vi "rd_data (Array of DBL).vi"(4 "record index":u32, 6 "record info":T3, 7 "recordLenFromStart":u64, 8 "error in (no error)":errorcluster, 9 "length":u64, 10 "record start":u64, 11 "ExcelRefnum":T4) -> (0 "error out":errorcluster, 2 "data_AllTypeData":T1, 3 "real length":u64)   [LabVIEW 2020, in "NI_ExcelFile.lvlib"]
uses:
  <vilib>/express/express shared/NI_ExcelFile/NI_ExcelFile.lvlib
  <vilib>/express/express shared/NI_ExcelFile/Ctrls/ExcelRefnum.ctl
  <vilib>/express/express shared/NI_ExcelFile/Ctrls/MainData.ctl
  <vilib>/express/express shared/NI_ExcelFile/Ctrls/StreamMode.ctl
  <vilib>/express/express shared/NI_ExcelFile/Ctrls/TimeColumnMode.ctl
  <vilib>/express/express shared/NI_ExcelFile/Ctrls/FileAttribute.ctl
  <vilib>/express/express shared/NI_ExcelFile/Ctrls/Columns.ctl
  <vilib>/express/express shared/NI_ExcelFile/Ctrls/ColumnInfo.ctl
  <vilib>/express/express shared/NI_ExcelFile/Ctrls/DataType.ctl
  <vilib>/express/express shared/NI_ExcelFile/Ctrls/wd_recordInfo.ctl
  <vilib>/express/express shared/NI_ExcelFile/Ctrls/disk_TemplateFile.ctl
  <vilib>/express/express shared/NI_ExcelFile/Ctrls/meta_file.ctl
  <vilib>/express/express shared/NI_ExcelFile/Ctrls/meta_Block.ctl
  <vilib>/express/express shared/NI_ExcelFile/Ctrls/meta_BlockType.ctl
  <vilib>/express/express shared/NI_ExcelFile/Ctrls/data_AllTypeData.ctl
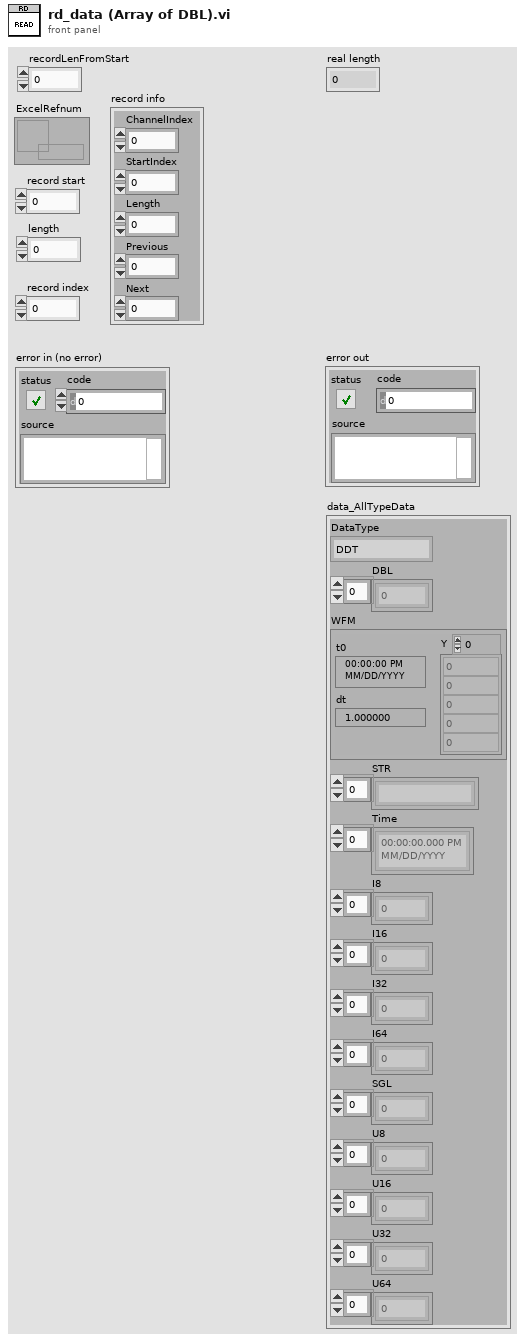
[diagram p1: front panel]
types:
  T1 = typedef "NI_ExcelFile.lvlib/data_AllTypeData.ctl" = cluster{"DataType":T2, "DBL":dbl[], "WFM":waveform(dbl), "STR":string[], "Time":timestamp[], "I8":i8[], "I16":i16[], "I32":i32[], "I64":i64[], "SGL":sgl[], "U8":u8[], "U16":u16[], "U32":u32[], "U64":u64[]}
  T2 = typedef "NI_ExcelFile.lvlib/DataType.ctl" = enum16{"DDT", "WFM", "Array of STR", "Array of DBL", "Array of I8", "Array of I16", "Array of I32", "Array of I64", "Array of SGL", "Array of U8", "Array of U16", "Array of U32", "Array of U64", "Array of Time"}
  T3 = typedef "NI_ExcelFile.lvlib/wd_recordInfo.ctl" = cluster{"ChannelIndex":u32, "StartIndex":u64, "Length":u64, "Previous":i32, "Next":i32}
  T4 = typedef "NI_ExcelFile.lvlib/ExcelRefnum.ctl" = refnum<data-value>
  T5 = typedef "NI_ExcelFile.lvlib/MainData.ctl" = cluster{"TargetFile":path, "StreamMode":T6, "Append?":bool, "ChunkSize":u64, "TimeColumnMode":T7, "TimestampFormat":string, "AbsoluteTime?":bool, "FileAttribute ":T8, "Column":T9, "FileRef":refnum<k1>, "MemoryRef":refnum<data-value>[], "RecordInfo":T3[], " ChannelPreviousInfo":u32[], "ChannelFirstRecord":u32[], "PredefinedFormattedValueLength":i64, "DiskTemplate":T11}
  T6 = typedef "NI_ExcelFile.lvlib/StreamMode.ctl" = enum16{"File", "Memory"}
  T7 = typedef "NI_ExcelFile.lvlib/TimeColumnMode.ctl" = enum16{"Empty", "OnePerCh", "One"}
  T8 = typedef "NI_ExcelFile.lvlib/FileAttribute.ctl" = cluster{"Creator":string, "Title":string, "SheetName":string}
  T9 = typedef "NI_ExcelFile.lvlib/Columns.ctl" = T10[]
  T10 = typedef "NI_ExcelFile.lvlib/ColumnInfo.ctl" = cluster{"Header":string, "Format":string, "DataType":T2, "Length":u64}
  T11 = typedef "NI_ExcelFile.lvlib/disk_TemplateFile.ctl" = cluster{"XMLRef":refnum<file>[], "ZipPath":path, "MetaFile":T12, "TempFolder":path}
  T12 = typedef "NI_ExcelFile.lvlib/meta_file.ctl" = cluster{"Ref":refnum<file>, "NextRow":i32, "NextPosition":i64, "Block":T13[]}
  T13 = typedef "NI_ExcelFile.lvlib/meta_Block.ctl" = cluster{"Version":u16, "Type":T14, "Length":i32, "Data":string}
  T14 = typedef "NI_ExcelFile.lvlib/meta_BlockType.ctl" = enum16{"NITag", "File", "Column"}
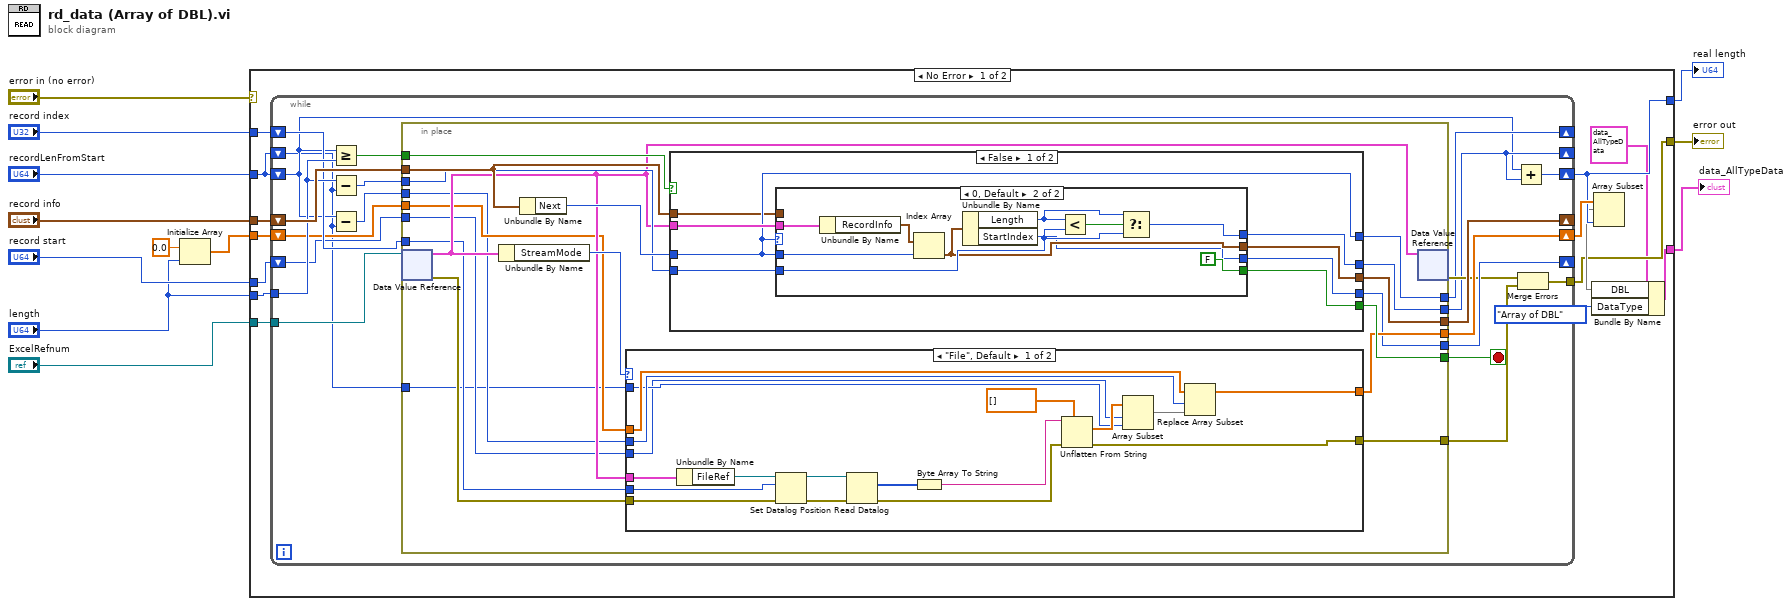
[diagram p0: block diagram]
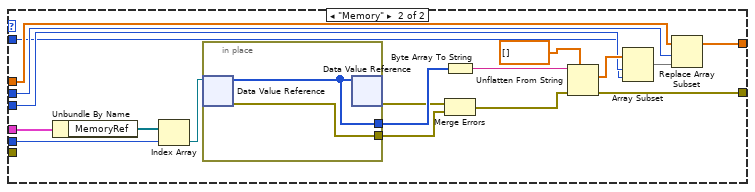
[diagram p2: hidden frame]
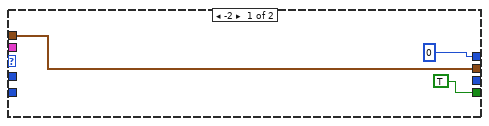
[diagram p3: hidden frame]
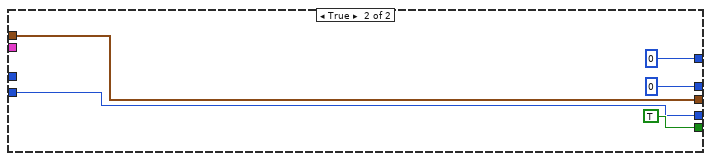
[diagram p4: hidden frame]
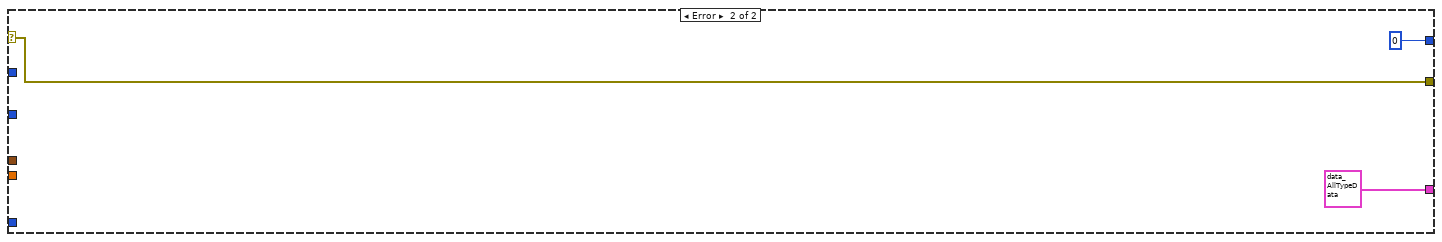
[diagram p5: hidden frame]
diagram:
  n1 = Initialize Array(0.0 ("element"), "length") -> (w3:dbl[])
  n2 = case shown="No Error" "error in (no error)" {
    selector: "error in (no error)" -> [_ w133]
    tunnel: w3 -> [w20 _]
    tunnel: [w15 w133] -> w12
    tunnel: "record start" -> [w26 _]
    tunnel: "record index" -> [w22 _]
    tunnel: "ExcelRefnum" -> [w25 _]
    tunnel: "recordLenFromStart" -> [w21 _]
    tunnel: "length" -> [w24 _]
    tunnel: "record info" -> [w23 _]
    tunnel: [w18 u64 0 ("recordLenFromStart")] -> w6
    tunnel: [w14 T1 {"DataType"=enum."DDT", "DBL"=[], "WFM"={"t0"=timestamp(0 s since 1904-01-01), "dt"=1.0, "Y"=[]}, "STR"=[], "Time"=[], "I8"=[], "I16"=[], "I32"=[], "I64"=[], "SGL"=[], "U8"=[], "U16"=[], "U32"=[], "U64"=[]} ("fmt_AllTypeData")] -> w1
    frame No Error {
      n3 = while {
        shift-right: [w30] -> _
        shift-left: w21 -> [w28]
        tunnel: w24 -> [w44]
        shift-right: [w45] -> _
        shift-left: w23 -> [w46]
        tunnel: w25 -> [w47]
        shift-right: [w42] -> w18
        shift-left: w21 -> [w29]
        shift-right: [w36] -> w19
        shift-left: w20 -> [w37]
        shift-right: [w31] -> _
        shift-left: w22 -> [w40]
        shift-right: [w35] -> _
        shift-left: w26 -> [w39]
        tunnel: [w32] -> w15
        stop <- w38 stop-if-true
        n4 = Greater Or Equal?(x=w29, y=w44) -> (x >= y?=w41:bool)
        n5 = Subtract(x=w44, y=w28) -> (x-y=w43:u64)
        n6 = Subtract(x=w29, y=w28) -> (x-y=w27:u64)
        n7 = in-place {
          in-place-border: w46 -> [w65]
          in-place-border: w28 -> [w48]
          in-place-border: [w63] -> w45
          in-place-border: w43 -> [w62]
          in-place-border: [w61] -> w30
          in-place-border: w41 -> [w60]
          in-place-border: w40 -> [w57]
          in-place-border: w39 -> [w56]
          in-place-border: [w55] -> w31
          in-place-border: [w54] -> w38
          in-place-border: w37 -> [w53]
          in-place-border: [w52] -> w36
          in-place-border: [w51] -> w35
          in-place-border: [w50] -> w33
          in-place-border: w27 -> [w49]
          n8 = in-place-dvr #1(w47) -> (w58:T5, w66:errorcluster)
          n9 = Unbundle By Name(w58) -> ("StreamMode"=w59:T6)
          n10 = Unbundle By Name(w65) -> ("Next"=w64:i32)
          n11 = case shown="\"File\", Default" w59 {
            tunnel: w57 -> [w81 w95]
            tunnel: w66 -> [w80 _]
            tunnel: w56 -> [w67 w92]
            tunnel: w58 -> [w83 w102]
            tunnel: w53 -> [w76 w100]
            tunnel: [w75 w99] -> w52
            tunnel: [w71 w90] -> w50
            tunnel: w49 -> [w69 w86]
            tunnel: w48 -> [w68 w85]
            frame "File", Default {
              n12 = Unbundle By Name(w83) -> ("FileRef"=w82:refnum<k1>)
              n13 = Set Datalog Position(4:w80, 6:w81, 7:w82) -> (0:w79:errorcluster, 3:w84:refnum<k1>)  [unwired: 1 in]
              n14 = Read Datalog(4:w79, 7:w84) -> (0:w72:errorcluster, 2:w78:u8[])  [unwired: 1 in, 1 out]
              n15 = Byte Array To String(unsigned byte array=w78) -> (string=w77:string)
              n16 = Unflatten From String(type=dbl[] [] ("Initial data"), binary string=w77, error in (no error)=w72) -> (value=w73:dbl[], error out=w71:errorcluster)  [unwired: 2 in, 1 out]
              n17 = Array Subset(array=w73, index=w67, length=w68) -> (w70:dbl[])
              n18 = Replace Array Subset(array=w76, new element=w70, index=w69) -> (w75:dbl[])
            }
            frame "Memory" {
              n19 = Unbundle By Name(w102) -> ("MemoryRef"=w96:refnum<data-value>[])
              n20 = Index Array(array=w96, index=w95) -> (element=w94:refnum<data-value>)
              n21 = in-place {
                in-place-border: [w104] -> w93
                in-place-border: [w103] -> w88
                n22 = in-place-dvr #2(w94) -> (w104:u8[], w103:errorcluster)
                n23 = in-place-dvr #2(w104) -> (w91:errorcluster)  [unwired: 1 out]
              }
              n24 = Byte Array To String(unsigned byte array=w93) -> (string=w101:string)
              n25 = Merge Errors(w91, w88) -> (w89:errorcluster)
              n26 = Unflatten From String(type=dbl[] [] ("Initial data"), binary string=w101, error in (no error)=w89) -> (value=w97:dbl[], error out=w90:errorcluster)  [unwired: 2 in, 1 out]
              n27 = Array Subset(array=w97, index=w92, length=w85) -> (w87:dbl[])
              n28 = Replace Array Subset(array=w100, new element=w87, index=w86) -> (w99:dbl[])
            }
          }
          n29 = case shown="False" w60 {
            tunnel: w65 -> [w107 w127]
            tunnel: w64 -> [w108 _]
            tunnel: [w109 w127] -> w63
            tunnel: w62 -> [w110 w126]
            tunnel: [w112 u64 0 ("Length")] -> w61
            tunnel: w58 -> [w111 _]
            tunnel: [w108 u32 0 ("next")] -> w55
            tunnel: [w106 TRUE] -> w54
            tunnel: [w105 w126] -> w51
            frame False {
              n30 = case shown="0, Default" w108 {
                tunnel: [u64 0 ("Length") w123] -> w112
                tunnel: w111 -> [_ w122]
                tunnel: w108 -> [_ w121]
                tunnel: w110 -> [_ w120]
                tunnel: [w115 w119] -> w109
                tunnel: w107 -> [w115 _]
                tunnel: [TRUE FALSE] -> w106
                tunnel: [_ w117] -> w105
                frame -2 {
                }
                frame 0, Default {
                  n31 = Unbundle By Name(w122) -> ("RecordInfo"=w125:T3[])
                  n32 = Index Array(array=w125, index=w121) -> (element=w119:T3)
                  n33 = Unbundle By Name(w119) -> ("Length"=w116:u64, "StartIndex"=w117:u64)
                  n34 = Less?(x=w116, y=w120) -> (x < y?=w124:bool)
                  n35 = Select(t=w116, s=w124, f=w120) -> (s? t:f=w123:u64)
                }
              }
            }
            frame True {
            }
          }
          n36 = in-place-dvr #1(w58) -> (w34:errorcluster)  [unwired: 1 out]
        }
        n37 = Add(x=w29, y=w30) -> (x+y=w42:u64)
        n38 = Merge Errors(w34, w33) -> (w32:errorcluster)
      }
      n39 = Array Subset(array=w19, length=w18) -> (w16:dbl[])  [unwired: 1 in]
      n40 = Bundle By Name(cluster=T1 {"DataType"=enum."DDT", "DBL"=[], "WFM"={"t0"=timestamp(0 s since 1904-01-01), "dt"=1.0, "Y"=[]}, "STR"=[], "Time"=[], "I8"=[], "I16"=[], "I32"=[], "I64"=[], "SGL"=[], "U8"=[], "U16"=[], "U32"=[], "U64"=[]} ("fmt_AllTypeData"), "DBL"=w16, "DataType"=DataType."Array of DBL") -> (w14:T1)
    }
    frame Error {
    }
  }
  "error out" <- w12
  "real length" <- w6
  "data_AllTypeData" <- w1
